vi "Configure Source.vi"(8 "error in (no error)":errorcluster, 10 "Source (F:Volt)":bool, 11 "E364x in":refnum<class "E364x.lvclass">) -> (0 "error out":errorcluster, 3 "E364x out":refnum<class "E364x.lvclass">)   [LabVIEW 2020, in "E364x.lvclass"]
uses:
  E364x.lvclass
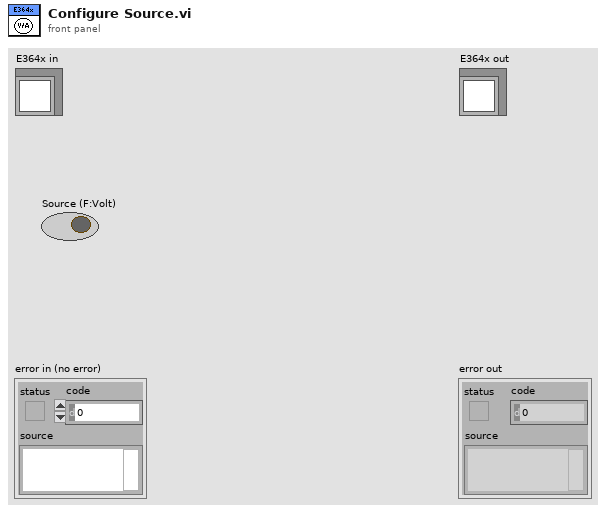
[diagram p1: front panel]
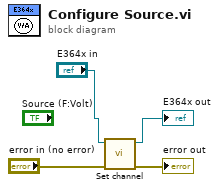
[diagram p0: block diagram]
diagram:
  n1 = call "Set channel.vi"("error in (no error)"="error in (no error)", "E364x in"="E364x in") -> ("error out"=→"error out":errorcluster, "E364x out"=→"E364x out":refnum<class "E364x.lvclass">)  [unwired: 7 in, 1 out]
